vi "Start.vi"(0 "reference in":refnum<class "niMmWave_Reciever.lvclass">, 5 "TX bursts":refnum<class "mmWave data.lvclass">[](array[class]), 7 "sequence":string[](array[string]), 9 "RX acq length":dbl=320000.0, 11 "error in (no error)":errorcluster) -> (4 "reference out":refnum<class "niMmWave_Reciever.lvclass">, 15 "error out":errorcluster)   [LabVIEW 2019, in "niMmWave_Reciever.lvclass"]
doc: "Starts insturment operation:"
uses:
  niMmWave_Reciever.lvclass
  C:/Barkhausen mmWave radar/Development/modules/mmw_instrument/src_LabVIEW/Host/SubVIs/mmWave instrument_class/mmWave instrument.lvclass
  mmWave data_class/mmWave data.lvclass
  mmWave instrument_class/Instrument state.ctl
  mmWave instrument_class/mmWave instrument.lvclass
  mmWave HW Control/mmWave HW Control.lvlib
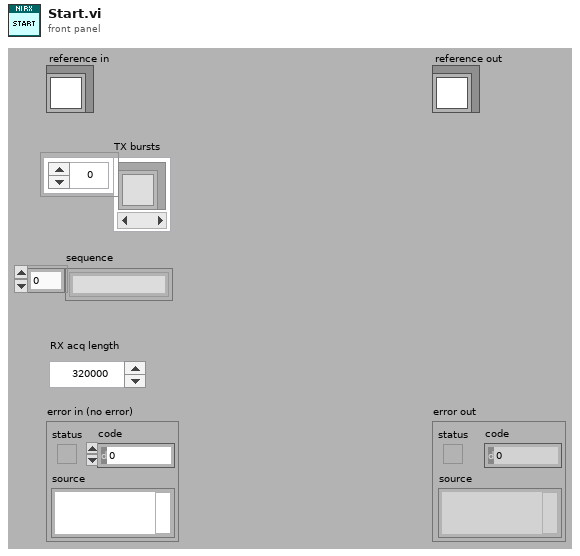
[diagram p1: front panel]
types:
  T1 = typedef "mmWave instrument.lvclass/Instrument state.ctl" = enum16{"Off", "Initialization", "Configuration", "Running", "Calibration"}
  T2 = typedef "mmWave instrument.lvclass/ObjectAttributes.ctl" = cluster{"mode":T3, "instr state":T1, "Max Fs":dbl, "Equalization coeff":cdb[], "LO sync en":bool, "Trig sync en":bool, "LO sources":T4, "LO Export":T5, "Fc.range":cluster{"min":dbl, "max":dbl}, "Sync mode":T6, "equalization en":bool, "sequence":string[]}
  T3 = typedef "mmWave instrument.lvclass/Instrument mode.ctl" = enum16{"RF", "IF", "BB"}
  T4 = typedef "mmWave HW Control.lvlib/LO sources.ctl" = cluster{"RX/LO1 src":string, "TX/LO1 src":string, "LO2 src":string}
  T5 = typedef "mmWave HW Control.lvlib/LO export.ctl" = cluster{"TX LO1 export":bool, "TX LO1 export level":dbl, "RX LO1 export":bool, "RX LO1 export level":dbl, "LO2 export":bool, "LO2 export level":dbl}
  T6 = typedef "mmWave instrument.lvclass/Sync mode.ctl" = enum16{"Slave", "Master"}
  T7 = typedef "niMmWave_Reciever.lvclass/ObjectAttributesRef.ctl" = refnum<data-value>
  T8 = typedef "niMmWave_Reciever.lvclass/ObjectAttributes.ctl" = cluster{"session":T9[], "HW.RX devices":T23, "RF config":T24, "RX trigger options":T25, "RX samples":i32, "RX Fs":dbl}
  T9 = typedef "Session.ctl" = cluster{"3620 session":refnum<queue>, "tx baseband session":T10, "rx baseband session":T18, "tx gain (dB)":dbl, "rx gain (dB)":dbl, "hardware configuration":T19, "gain ranging":T21[], "pxi trigger bus information":T22}
  T10 = typedef "Tx Baseband Session.ctl" = cluster{"3610 session":T11, "7902 reference":T17}
  T11 = typedef "ni3610_and_ni3630_Driver_Lib.lvlib/Main Settings.ctl" = cluster{"VISA resource name":refnum<visa-resource-name>, "Address Space":T12, "window_offset":u32, "register_addresses":T13, "required_MM_fpga_version":cluster{"signature":u32, "hardware":u32, "current revision":u32, "oldest revision":u32}, "CPLD Oldest Compat Version ":cluster{"hardware":u32, "CPLD firmware":u32}, "MM_FPGA_image_location":string, "is_init":bool, "card_type":T14, "DacLmkConfigFileName":string, "AdcLmkConfigFileName":string, "AdcConfigFileName":string, "DacConfigFileName_RevA":string, "DacConfigFileName_RevB":string, "Mulde hardware revision":u8, "bypass DAC PLL\n":bool, "IQ Card Revision":T15, "board capability":T16}
  T12 = typedef "VISA Register Access Address Space.ctl" = u16
  T13 = typedef "ni3610_and_ni3630_Driver_Lib.lvlib/Register Adresses.ctl" = cluster{"MM based Registers":cluster{"Revision":u32, "OldestCompatRev":u32, "signature":u32, "scratch":u32, "LedControl":u32, "BoardHwRev":u32, "BoardControl":u32, "ThermalStatus":u32, "BasebandStatus":u32, "BasebandControl":u32, "BasebandAuxSetup":u32, "BasebandAuxStatus":u32, "LmkSyncOutSetup":u32, " AdcSyncOutSetup":u32, " InjSyncOutSetup":u32, " PxiTrig0OutSetup":u32, " PxiTrig1OutSetup":u32, " PxiTrig2OutSetup":u32, " PxiTrig3OutSetup":u32, " PxiTrig4OutSetup":u32, " PxiTrig5OutSetup":u32, " PxiTrig6OutSetup":u32, " PxiTrig7OutSetup":u32}, "CPLD based Registers":cluster{"SlaveSignature":u32, "SlaveRevision":u32, "SlaveOldestCompatRev":u32, "SlaveScratch":u32, "SlaveSetup":u32, "SlaveStatus":u32, "IDacReg_offset":u32, "LMKRegGrp0_offset":u32, "QDacReg_offset":u32, "BrdTempSensorVal":u32, "TempSensorPowerDown":u32, "GPIOReg_offset":u32, "IAdcReg_offset":u32, "QAdcReg_offset":u32, "LMKRegGrp1_offset":u32, "QadcTempSensorVal":u32, "IadcTempSensorVal":u32, "RevisionReg":u32, "VcxoReg":u32, "CpldStatusReg":u32, "PowerReg":u32, "VBiasEnReg":u32, "ExtRefOeReg":u32, "QdacCtrlReg":u32, "QdacStatusReg":u32, "IdacCtrlReg":u32, "IdacStatusReg":u32, "QdacJtagIn":u32, "QdacJtagOut":u32, "IdacJtagIn":u32, "IdacJtagOut":u32, "IqDcSetupReg":u32, "QadcStatusReg":u32, "IadcStatusReg":u32, "BrdSetupReg":u32, "IqDcRevisionReg":u32, "PllStatusReg":u32, "EndpointScratchReg":u32, "AdcSyncCfgReg":u32, "IqCardOpampReg":u32}, "CPLD Register Offset":u32, "MM  Register Offset":u32, " PxiTrig0OutSetup":u32}
  T14 = typedef "ni3610_and_ni3630_Driver_Lib.lvlib/Base Card Type.ctl" = enum16{"unspecified", "ADC", "DAC"}
  T15 = typedef "ni3610_and_ni3630_Driver_Lib.lvlib/IQ Card Revision.ctl" = enum16{"RevA", "RevB", "RevC", "RevD"}
  T16 = typedef "ni3610_and_ni3630_Driver_Lib.lvlib/Board Capability.ctl" = cluster{"baseband sync":enum16{"no baseband sync", "baseband sync"}}
  T17 = typedef "Blank FPGA Reference.ctl" = refnum<k20>
  T18 = typedef "Rx Baseband Session.ctl" = cluster{"3630 session":T11, "7902 reference":T17}
  T19 = typedef "Hardware Configuration.ctl" = cluster{"direction":T20, "baseband only":bool}
  T20 = typedef "Direction.ctl" = enum16{"Transceiver", "Receiver", "Transmitter"}
  T21 = typedef "Gain Ranging.ctl" = cluster{"gain ranging active scope":string, "gain ranging stream session":refnum<k20>}
  T22 = typedef "PXI Trigger Bus Info.ctl" = cluster{"chassis resource name":refnum<visa-resource-name>, "7902R (TX)":i16, "3610 (TX)":i16, "3620 (IF)":i16, "3630 (RX)":i16, "7902R (RX)":i16}
  T23 = typedef "mmWave HW Control.lvlib/HW RX resources cluster.ctl" = cluster{"HW.IF":tag, "HW.ADC":refnum<visa-resource-name>, "HW.RX FPGA":tag}
  T24 = typedef "mmWave HW Control.lvlib/HW RX RF config cluster.ctl" = cluster{"Gain":dbl, "Frequency":dbl, "mmWave adapter":string}
  T25 = typedef "TX trigger config.ctl" = cluster{"delay":dbl, "trig source":T26, "PXI src":i32, "export":T27, "PXI dest":i32}
  T26 = typedef "FPGA Utility.lvlib/FPGA driver trigger source.ctl" = enum16{"Use Tclk", "PXI_Trig", "Aurora RX trig"}
  T27 = typedef "FPGA Utility.lvlib/FPGA driver trigger destination.ctl" = enum16{"None", "Source trig", "Synced trig", "Delayed sync"}
  T28 = typedef "Constants.ctl" = cluster{"data clock rate (Hz)":dbl, "sample rate (Hz)":dbl, "sample rate selector string":string, "default tx bitfile path":path, "default rx bitfile path":path, "default proc bitfile path":path}
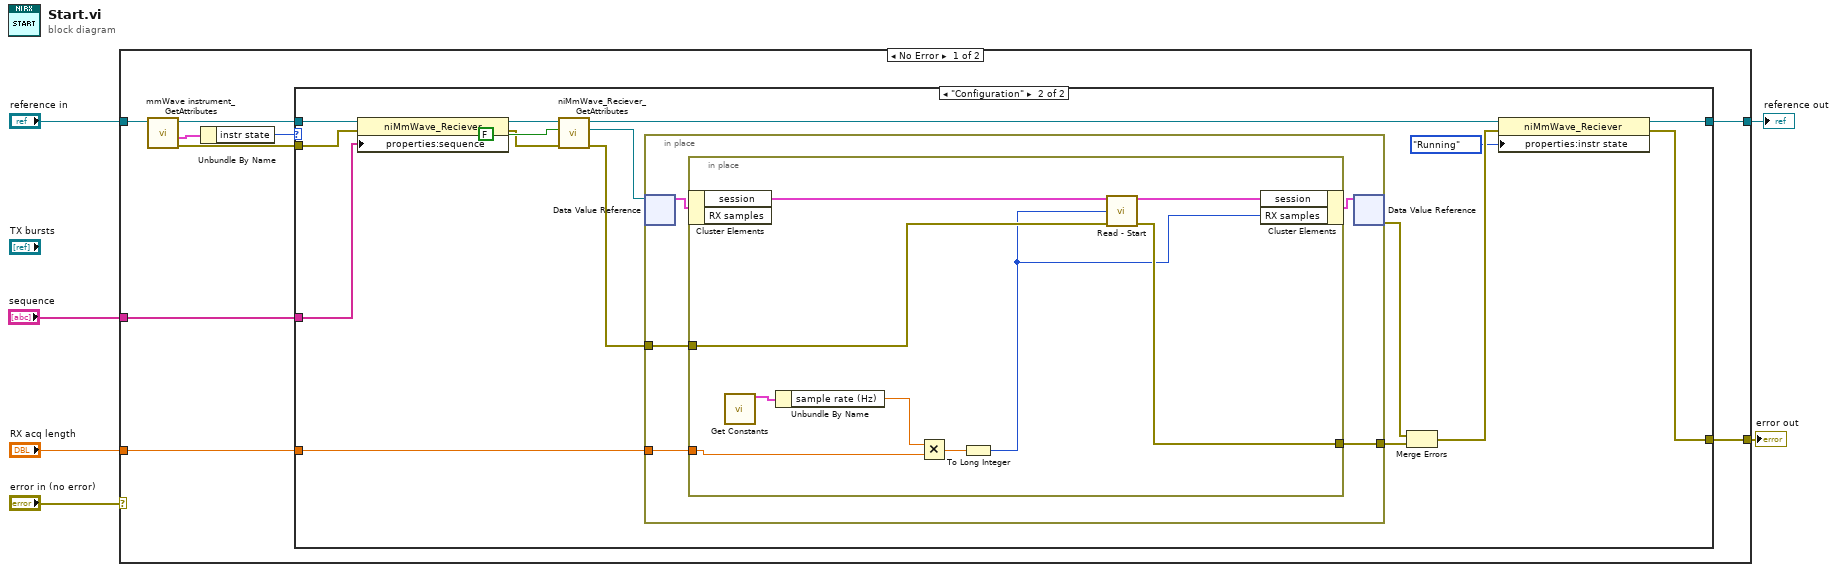
[diagram p0: block diagram]
diagram:
  n1 = case shown="No Error" "error in (no error)" {
    selector: "error in (no error)" -> [_ w48]
    tunnel: [w15 w48] -> w5
    tunnel: [w13 w47] -> w3
    tunnel: "reference in" -> [w14 w47]
    tunnel: "RX acq length" -> [w8 _]
    tunnel: "sequence" -> [w7 _]
    frame No Error {
      n2 = call "mmWave instrument_GetAttributes.vi"("reference in"=w14) -> ("error out"=w9:errorcluster, "attributes"=w11:T2, "reference out"=w12:refnum<class "niMmWave_Reciever.lvclass">)  [unwired: 7 in, 1 out]
      n3 = Unbundle By Name(w11) -> ("instr state"=w10:T1)
      n4 = case shown="\"Configuration\"" w10 {
        tunnel: [_ w22] -> w15
        tunnel: [w16 w25] -> w13
        tunnel: w12 -> [w16 w28]
        tunnel: w9 -> [_ w19]
        tunnel: w8 -> [_ w27]
        tunnel: w7 -> [_ w18]
        frame "Off", Default {
        }
        frame "Configuration" {
          n5 = property class="niMmWave_Reciever"(reference=w28, error in=w19, "properties:sequence"=w18) -> (reference out=w20:refnum<class "niMmWave_Reciever.lvclass">, error out=w17:errorcluster)
          n6 = call "niMmWave_Reciever_GetAttributes.vi"("error in (no error)"=w17, "return data? (T)"=FALSE, "reference in"=w20) -> ("error out"=w21:errorcluster, "attributes ref"=w29:T7, "reference out"=w30:refnum<class "niMmWave_Reciever.lvclass">)  [unwired: 5 in, 1 out]
          n7 = in-place {
            in-place-border: w27 -> [w35]
            in-place-border: w21 -> [w34]
            in-place-border: [w33] -> w26
            n8 = in-place-dvr #1(w29) -> (w36:T8)  [unwired: 1 out]
            n9 = in-place {
              in-place-border: w35 -> [w41]
              in-place-border: w34 -> [w44]
              in-place-border: [w43] -> w33
              n10 = in-place-cluster #2(w36) -> ("session"=w46:T9[])  [unwired: 1 out]
              n11 = call "Get Constants.vi"() -> ("constants"=w39:T28)  [unwired: 15 in]
              n12 = Unbundle By Name(w39) -> ("sample rate (Hz)"=w38:dbl)
              n13 = Multiply(x=w38, y=w41) -> (x*y=w42:dbl)
              n14 = To Long Integer(number=w42) -> (32bit integer=w40:i32)
              n15 = call "Read - Start.vi"("session in"=w46, "number of samples"=w40, "error in"=w44) -> ("session out"=w45:T9[], "error out"=w43:errorcluster)  [unwired: 11 in]
              n16 = in-place-cluster #2("session"=w45, "RX samples"=w40) -> (w37:T8)
            }
            n17 = in-place-dvr #1(w37) -> (w32:errorcluster)  [unwired: 1 out]
          }
          n18 = Merge Errors(w32, w26) -> (w24:errorcluster)
          n19 = property class="niMmWave_Reciever"(reference=w30, error in=w24, "properties:instr state"=Instrument_state."Running" ("instr state")) -> (reference out=w25:refnum<class "niMmWave_Reciever.lvclass">, error out=w22:errorcluster)
        }
      }
    }
    frame Error {
    }
  }
  "error out" <- w5
  "reference out" <- w3
